vi "pp2_log_toString_trial.vi"(11 "Trial in":T1={"Trial Type Number"=1, "Trial Type"=enum."GO", "Trial Weight"=100, "Shock (mA)"=0.3, "Duration (ms)"=0.25, "Sound Type"=enum."04 FM Sweep", "Stim P1"=4000.0, "Stim P2"=0.0, "Stim P3"=0.0, "Stim P4"=2000.0, "DAQ Amplitude (V)"=0.25} {"DAQ Amplitude (V)" min=0.0 max=5.0 format="%_6g"; "Shock (mA)" min=-1.0 max=5.0; "Trial Weight" step=1; "Duration (ms)" min=0.0 max=1.0; "Trial Type Number" min=1 max=256 step=1}) -> (0 "TRIALMEMO String":string, 3 "spreadsheet string":string)   [LabVIEW 2013]
uses:
  LV3/impl/pp3_CTL_Trial.ctl
  LV3/impl/pp3_CTL_TrialType.ctl
  labolabo2/waveforms/WFTypes.ctl
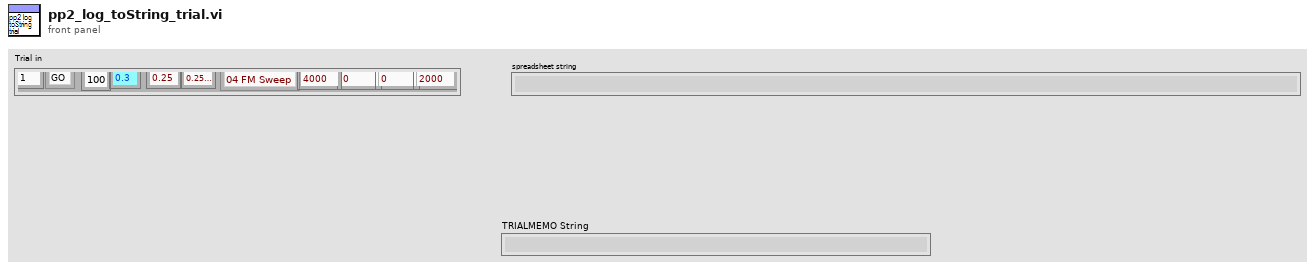
[diagram p1: front panel]
types:
  T1 = typedef "pp3_CTL_Trial.ctl" = cluster{"Trial Type Number":i16, "Trial Type":T2, "Trial Weight":u32, "Shock (mA)":dbl, "Duration (ms)":dbl, "Sound Type":T3, "Stim P1":dbl, "Stim P2":dbl, "Stim P3":dbl, "Stim P4":dbl, "DAQ Amplitude (V)":dbl}
  T2 = typedef "pp3_CTL_TrialType.ctl" = enum16{"OFF", "GO", "NOGO", "TEST"}
  T3 = typedef "WFTypes.ctl" = enum16{"00 NULL", "01 DC", "02 Noise", "03 Pure Tone", "04 FM Sweep"}
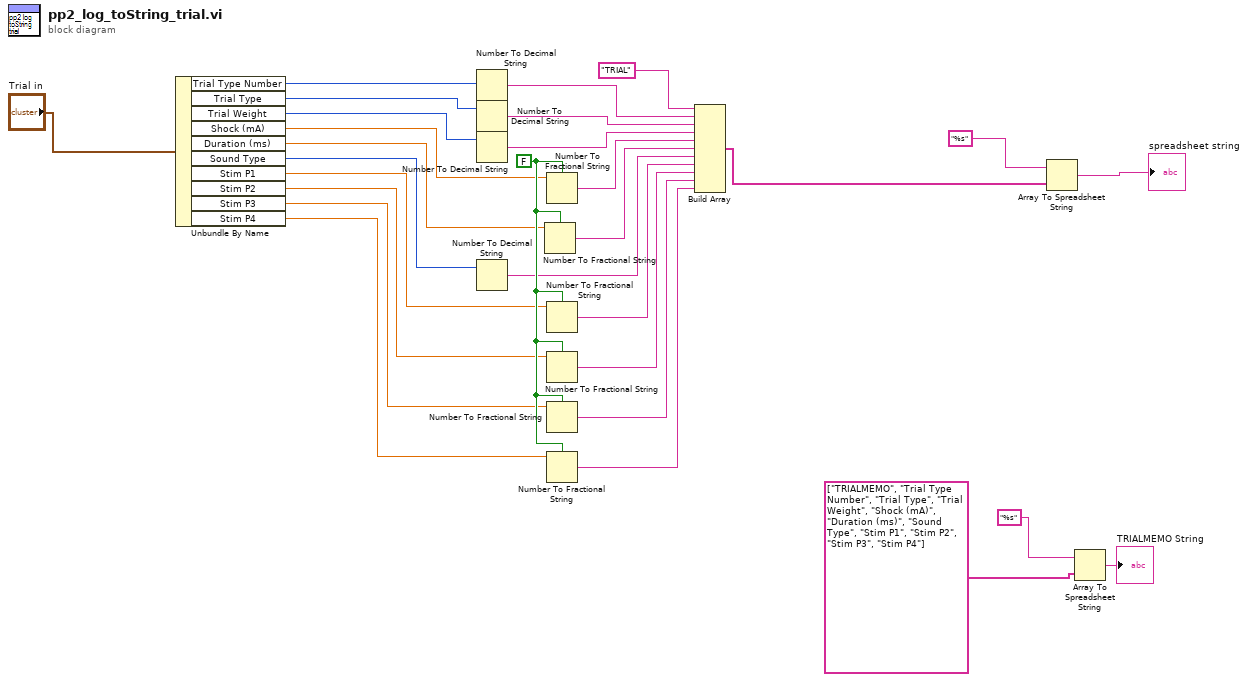
[diagram p0: block diagram]
diagram:
  w18 = FALSE
  n1 = Unbundle By Name("Trial in") -> ("Trial Type Number"=w22:i16, "Trial Type"=w21:T2, "Trial Weight"=w20:u32, "Shock (mA)"=w10:dbl, "Duration (ms)"=w9:dbl, "Sound Type"=w19:T3, "Stim P1"=w8:dbl, "Stim P2"=w7:dbl, "Stim P3"=w6:dbl, "Stim P4"=w5:dbl)
  n2 = Number To Decimal String(number=w22) -> (decimal integer string=w24:string)  [unwired: 1 in]
  n3 = Number To Decimal String(number=w21) -> (decimal integer string=w29:string)  [unwired: 1 in]
  n4 = Number To Decimal String(number=w20) -> (decimal integer string=w28:string)  [unwired: 1 in]
  n5 = Number To Decimal String(number=w19) -> (decimal integer string=w15:string)  [unwired: 1 in]
  n6 = Number To Fractional String(use system decimal point (T)=w18, number=w9) -> (F-format string=w16:string)  [unwired: 2 in]
  n7 = Number To Fractional String(use system decimal point (T)=w18, number=w10) -> (F-format string=w17:string)  [unwired: 2 in]
  n8 = Number To Fractional String(use system decimal point (T)=w18, number=w8) -> (F-format string=w14:string)  [unwired: 2 in]
  n9 = Number To Fractional String(use system decimal point (T)=w18, number=w7) -> (F-format string=w13:string)  [unwired: 2 in]
  n10 = Number To Fractional String(use system decimal point (T)=w18, number=w6) -> (F-format string=w12:string)  [unwired: 2 in]
  n11 = Number To Fractional String(use system decimal point (T)=w18, number=w5) -> (F-format string=w11:string)  [unwired: 2 in]
  n12 = Build Array("TRIAL" ("element"), w24, w29, w28, w17, w16, w15, w14, w13, w12, w11) -> (w26:string[])
  n13 = Array To Spreadsheet String(array=w26, 3:"%s" ("format string")) -> (spreadsheet string=→"spreadsheet string":string)  [unwired: 1 in]
  n14 = Array To Spreadsheet String(array=string[] ["TRIALMEMO", "Trial Type Number", "Trial Type", "Trial Weight", "Shock (mA)", "Duration (ms)", "Sound Type", "Stim P1", "Stim P2", "Stim P3", "Stim P4"], 3:"%s" ("format string")) -> (spreadsheet string=→"TRIALMEMO String":string)  [unwired: 1 in]
